vi "To File.vi"(6 "Replace? [T]":bool=TRUE, 7 "Persitant only? [T]":bool=TRUE, 8 "error in (no error)":errorcluster, 10 "Path [Paths]":path, 11 "Carya Config in":refnum<class "Carya Config.lvclass">) -> (0 "error out":errorcluster, 3 "Carya Config out":refnum<class "Carya Config.lvclass">)   [LabVIEW 2013, in "Carya Config.lvclass"]
doc: "Copyright 2018, Carya Automatisering, Wiebe Walstra."
uses:
  Carya Config.lvclass
  Carya Config.lvclass/Carya Config.ctl
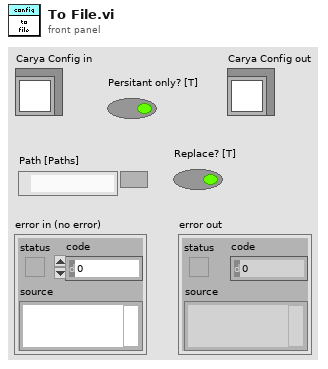
[diagram p1: front panel]
types:
  T1 = enum16{"open", "replace", "create", "open or create", "replace or create", "replace or create with confirmation"}
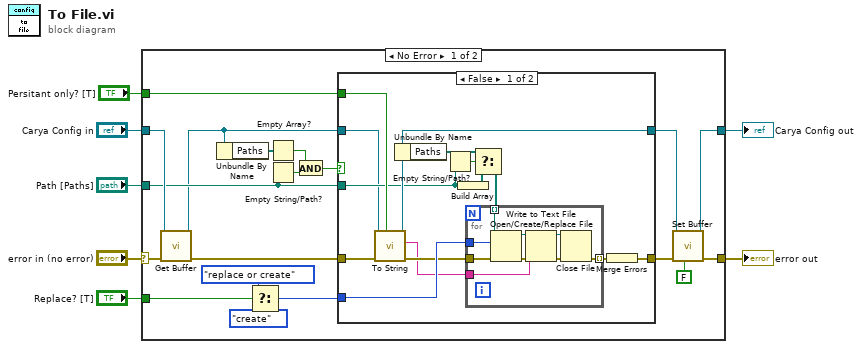
[diagram p0: block diagram]
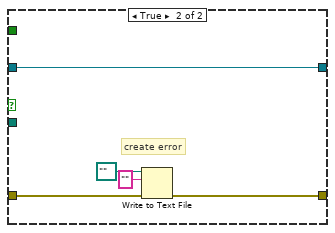
[diagram p2: hidden frame]
diagram:
  n1 = case shown="No Error" "error in (no error)" {
    selector: "error in (no error)" -> [w26 w56]
    tunnel: [w20 w56] -> w6
    tunnel: [w19 w55] -> w4
    tunnel: "Carya Config in" -> [w21 w55]
    tunnel: "Path [Paths]" -> [w14 _]
    tunnel: "Replace? [T]" -> [w25 _]
    tunnel: "Persitant only? [T]" -> [w17 _]
    frame No Error {
      n2 = call-dynamic "Get Buffer.vi"("error in (no error)"=w26, "Carya Config in"=w21) -> ("error out"=w18:errorcluster, "Config"=w13:refnum<class "Carya Config.lvclass">)  [unwired: 8 in]
      n3 = Unbundle By Name(w13) -> ("Paths"=w12:path[])
      n4 = Select(t=T1."replace or create" ("operation (0:open)"), s=w25, f=T1."create") -> (s? t:f=w22:T1)
      n5 = Empty Array?(array=w12) -> (empty?=w10:bool)
      n6 = Empty String/Path?(string/path=w14) -> (empty?=w11:bool)
      n7 = And(x=w10, y=w11) -> (x .and. y?=w9:bool)
      n8 = case shown="False" w9 {
        tunnel: w22 -> [w36 _]
        tunnel: w18 -> [w35 w53]
        tunnel: w17 -> [w33 _]
        tunnel: [w30 w52] -> w16
        tunnel: [w29 w54] -> w15
        tunnel: w14 -> [w28 _]
        tunnel: w13 -> [w27 w54]
        frame False {
          n9 = call-dynamic "To String.vi"("Persitant only? [T]"=w33, "error in (no error)"=w35, "Carya Config in"=w27) -> ("error out"=w34:errorcluster, "String"=w32:string, "Carya Config out"=w29:refnum<class "Carya Config.lvclass">)  [unwired: 6 in]
          n10 = Unbundle By Name(w29) -> ("Paths"=w38:path[])
          n11 = Empty String/Path?(string/path=w28) -> (empty?=w39:bool)
          n12 = Build Array(w28) -> (w31:path[])
          n13 = Select(t=w38, s=w39, f=w31) -> (s? t:f=w37:path[])
          n14 = for {
            tunnel: [w49] -> w40 mode=indexing
            tunnel: w37 -> [w48] mode=indexing
            tunnel: w36 -> [w47]
            tunnel: w34 -> [w46]
            tunnel: w32 -> [w45]
            n15 = Open/Create/Replace File(file path (use dialog)=w48, error in=w46, operation (0:open)=w47) -> (refnum out=w43:refnum<file>, error out=w41:errorcluster)  [unwired: 3 in, 1 out]
            n16 = Write to Text File(file (use dialog)=w43, text=w45, error in=w41) -> (refnum out=w42:refnum<file>, error out=w44:errorcluster)  [unwired: 1 in, 1 out]
            n17 = Close File(refnum=w42, error in=w44) -> (error out=w49:errorcluster)  [unwired: 1 out]
          }
          n18 = Merge Errors(w40) -> (w30:errorcluster)
        }
        frame True {
          # "create error"
          n19 = Write to Text File(file (use dialog)=path "", text="", error in=w53) -> (error out=w52:errorcluster)  [unwired: 1 in, 2 out]
        }
      }
      n20 = call-dynamic "Set Buffer.vi"("Set? [T]"=FALSE, "error in (no error)"=w16, "Carya Config"=w15) -> ("error out"=w20:errorcluster, "Carya Config out"=w19:refnum<class "Carya Config.lvclass">)  [unwired: 7 in]
    }
    frame Error {
    }
  }
  "error out" <- w6
  "Carya Config out" <- w4
